vi "Agilent SNA Set Measurement.vi"(4 "Trace":i8=1 min=1 max=99 step=1, 5 "Parameter":T1 {"Stimulus Port" min=1 step=1; "Response Port" min=1 step=1}, 6 "Channel":i8=1 min=1 max=99 step=1, 7 "Agilent SNA & SWP":T2, 8 "error in (no error)":errorcluster, 10 "Measurement (SXX)":T4=enum."Analog In - Aux In", 11 "VISA Resource Names":T3) -> (0 "error out":errorcluster, 3 "dup VISA Resource Names":T3)   [LabVIEW 2011]
doc: "This VI for the HP8753B Network Analyzer sets the measurement."
uses:
  TypeDefs/Agilent SNA Measurement.ctl
  TypeDefs/Agilent SNA VISA.ctl
  TypeDefs/Agilent SNA Instrument Info.ctl
  tests/S Parameter/TypeDefs/SP Parameter.ctl
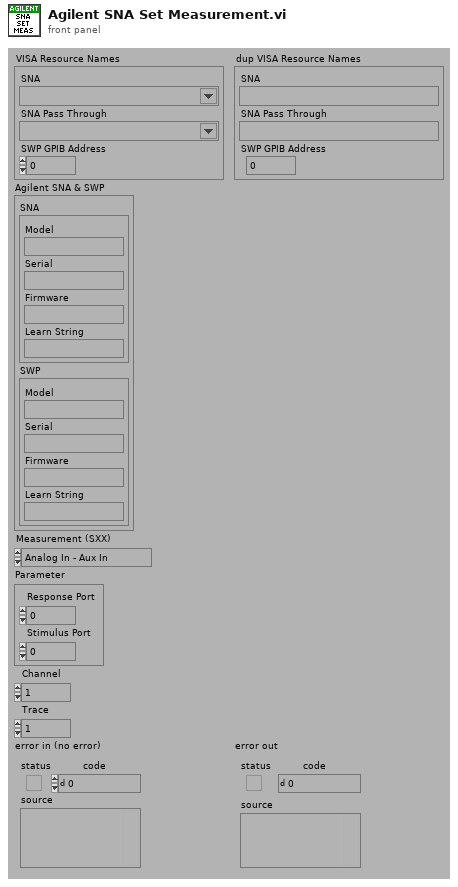
[diagram p1: front panel]
types:
  T1 = typedef "SP Parameter.ctl" = cluster{"Stimulus Port":i8, "Response Port":i8}
  T2 = typedef "Agilent SNA Instrument Info.ctl" = cluster{"SNA":cluster{"Model":string, "Serial":string, "Firmware":string, "Learn String":string}, "SWP":cluster{"Model":string, "Serial":string, "Firmware":string, "Learn String":string}}
  T3 = typedef "Agilent SNA VISA.ctl" = cluster{"SNA":refnum<visa-resource-name>, "SNA Pass Through":refnum<visa-resource-name>, "SWP GPIB Address":i32}
  T4 = typedef "Agilent SNA Measurement.ctl" = enum32{"SXX", "A", "B", "C", "R", "A/B", "A/C", "A/R", "B/A", "B/C", "B/R", "C/A", "C/B", "C/R", "R/A", "R/B", "R/C", "Analog In - Aux In"}
  T5 = typedef "Agilent SNA Model.ctl" = enum16{"Not Supported", "8757X"}
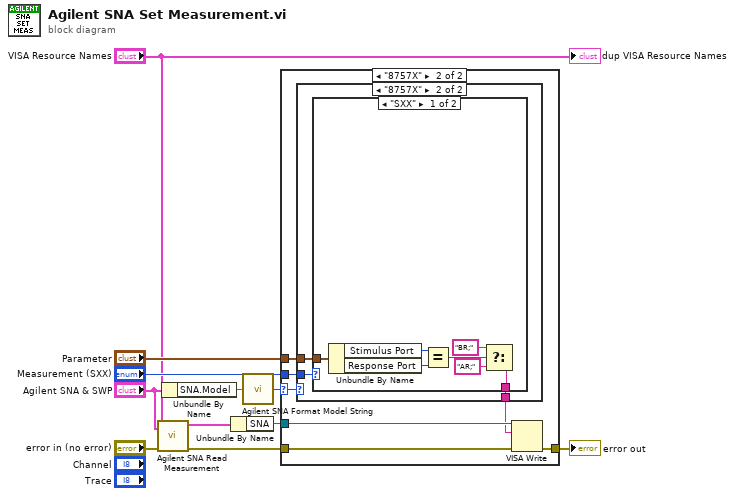
[diagram p0: block diagram]
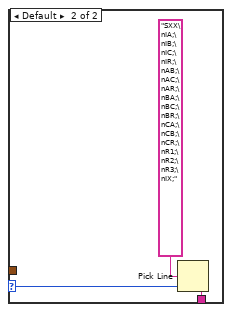
[diagram p4: hidden frame]
diagram:
  n1 = call "Agilent SNA Read Measurement.vi"("Agilent SNA & SWP"="Agilent SNA & SWP", "error in (no error)"="error in (no error)", "VISA Resource Names"="VISA Resource Names") -> ("error out"=w10:errorcluster, "dup VISA Resource Names"=w3:T3)  [unwired: 1 in, 6 out]
  n2 = Unbundle By Name("Agilent SNA & SWP") -> ("SNA.Model"=w7:string)
  n3 = Unbundle By Name(w3) -> ("SNA"=w2:refnum<visa-resource-name>)
  n4 = call "Agilent SNA Format Model String.vi"("Model String"=w7) -> ("Model"=w4:T5)
  n5 = case shown="\"8757X\"" w4 {
    selector: w4 -> [_ w16]
    tunnel: w10 -> [w12 w19]
    tunnel: "Measurement (SXX)" -> [_ w18]
    tunnel: "Parameter" -> [_ w15]
    tunnel: [w12 w17] -> w5
    tunnel: w2 -> [_ w14]
    frame "Not Supported" {
    }
    frame "8757X" {
      n6 = case shown="\"8757X\"" w16 {
        tunnel: w18 -> [_ w22]
        tunnel: w15 -> [_ w21]
        tunnel: [_ w20] -> w13
        frame "Not Supported" {
        }
        frame "8757X" {
          n7 = case shown="\"SXX\"" w22 {
            selector: w22 -> [_ w30]
            tunnel: [w23 w31] -> w20
            tunnel: w21 -> [w29 _]
            frame "SXX" {
              n8 = Unbundle By Name(w29) -> ("Stimulus Port"=w28:i8, "Response Port"=w27:i8)
              n9 = Equal?(x=w28, y=w27) -> (x = y?=w26:bool)
              n10 = Select(t="BR;", s=w26, f="AR;") -> (s? t:f=w23:string)
            }
            frame Default {
              n11 = Pick Line(multi-line string="SXX\nIA;\nIB;\nIC;\nIR;\nAB;\nAC;\nAR;\nBA;\nBC;\nBR;\nCA;\nCB;\nCR;\nR1;\nR2;\nR3;\nIX;", line index=w30) -> (output string=w31:string)  [unwired: 1 out]
            }
          }
        }
      }
      n12 = VISA Write(VISA resource name=w14, write buffer=w13, error in (no error)=w19) -> (error out=w17:errorcluster)  [unwired: 2 out]
    }
  }
  "error out" <- w5
  "dup VISA Resource Names" <- "VISA Resource Names"
